vi "Test All.vi"(11 "Error in":errorcluster) -> (15 "Error out":errorcluster)   [LabVIEW 2020, in "CelsiusToFarenheitTests.lvlib"]
doc: "This vi runs all the test cases for the Celsius to Fahrenheit assignment. Also the test report gets saved as a xml format.\n\n* USES *\nDrona, G-CLI and Caraya"
uses:
  CelsiusToFarenheitTests.lvlib
  <vilib>/addons/_JKI Toolkits/Caraya/classes/Test Suite/Define Test Suite (JUnit Report).vi
  <vilib>/addons/_JKI Toolkits/Caraya/classes/Test Suite/Test Suite.lvclass
  <vilib>/addons/_JKI Toolkits/Caraya/classes/Test/Test.lvclass
  <vilib>/Wiresmith Technology/G CLI/CLI Class/CLI.lvclass
panel:
  # "TESTING ALL TEST CASES FOR CELSIUS TO FAHRENHEIT"
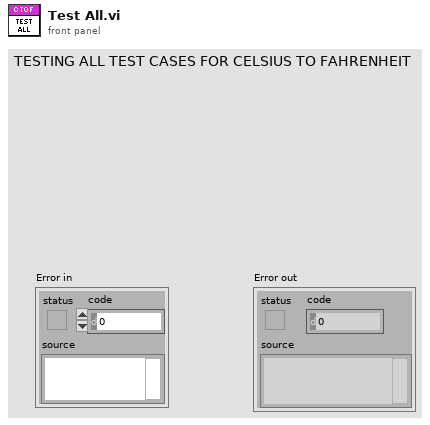
[diagram p1: front panel]
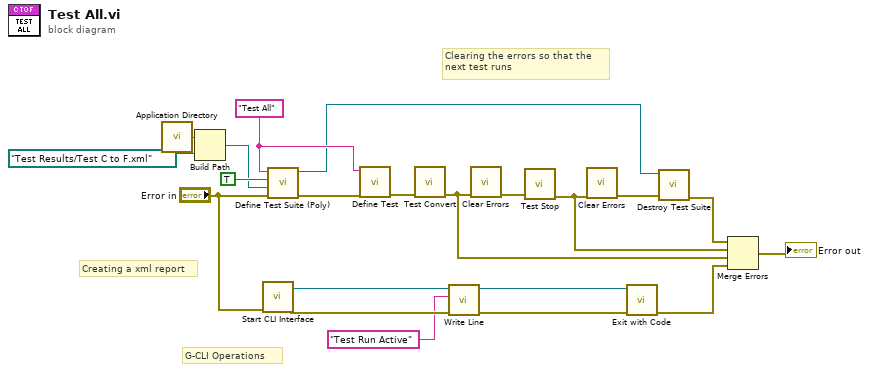
[diagram p0: block diagram]
diagram:
  w16 = "Test All" ("Label (VI Title)")
  # "G-CLI Operations"
  # "Creating a xml report"
  # "Clearing the errors so that the\nnext test runs"
  n1 = call <vilib>:"Application Directory.vi"() -> ("Application Directory"=w21:path)
  n2 = Build Path(base path=w21, name or relative path=path "Test Results/Test C to F.xml") -> (appended path=w18:path)
  n3 = call <vilib>:"Start CLI Interface.vi"("error in (no error)"="Error in") -> ("error out"=w6:errorcluster, "CLI out"=w4:refnum<class "CLI.lvclass">)  [unwired: 7 in, 2 out]
  n4 = call-poly <vilib>:"Define Test Suite (Poly).vi"("error in (no error)"="Error in", "Report Path"=w18, "Interactive"=TRUE, "Label (VI Title)"=w16) -> ("error out"=w17:errorcluster, "Test Suite"=w15:refnum<class "Test Suite.lvclass">)  [unwired: 6 in]
  n5 = call <vilib>:"Define Test.vi"("error in (no error)"=w17, "Label (VI Title)"=w16) -> ("error out"=w14:errorcluster)  [unwired: 9 in]
  n6 = call "Test Convert.vi"("Error in"=w14) -> ("Error out"=w10:errorcluster)  [unwired: 14 in]
  n7 = call <vilib>:"Write Line.vi"("error in (no error)"=w6, "Text to Write"="Test Run Active", "CLI in"=w4) -> ("error out"=w3:errorcluster, "CLI out"=w2:refnum<class "CLI.lvclass">)  [unwired: 7 in]
  n8 = call <vilib>:"Clear Errors.vi"("error in (no error)"=w10) -> ("error out"=w13:errorcluster)  [unwired: 5 in, 1 out]
  n9 = call "Test Stop.vi"("Error in"=w13) -> ("Error out"=w9:errorcluster)  [unwired: 14 in]
  n10 = call <vilib>:"Clear Errors.vi"("error in (no error)"=w9) -> ("error out"=w11:errorcluster)  [unwired: 5 in, 1 out]
  n11 = call <vilib>:"Exit with Code.vi"("error in (no error)"=w3, "CLI in"=w2) -> ("error out"=w1:errorcluster)  [unwired: 9 in]
  n12 = call-dynamic "Destroy Test Suite.vi"("error in (no error)"=w11, "Test Suite in"=w15) -> ("error out"=w12:errorcluster)  [unwired: 8 in, 1 out]
  n13 = Merge Errors(w12, w9, w10, w1) -> (→"Error out":errorcluster)
